vi "Agilent SNA Read Status Bytes.vi"(7 "Agilent SNA & SWP":T1, 8 "error in (no error)":errorcluster, 11 "VISA Resource Names":T2) -> (0 "error out":errorcluster, 1 "Extended Status Byte":bool[](array[boolean]), 2 "Status Byte":bool[](array[boolean]), 3 "dup VISA Resource Names":T2)   [LabVIEW 2011]
doc: "This VI for the HP8753B Network Analyzer reads the status byte and the two event status registers. The two status registers are read out as regular output and will therefore clear anything already in the output queue."
uses:
  TypeDefs/Agilent SNA VISA.ctl
  TypeDefs/Agilent SNA Instrument Info.ctl
panel:
  # "Self Test Failure\n\nOperation Failure\n\nKnob Activity\n\nAction Requested Not Possible\n\nLimit Test Failed\n\nFront Panel Preset or Power On\n\nDetector Uncal"
  # "Any Front Panel Key Pressed\n\nNumeric Entry Completed\n\nChange in Extended Status Byte\n\nSoftkey Only Pressed\n\nOperation Complete\n\nHP-IB Syntax Error\n\nRequest Service (SRQ)\n\nSweep Complete"
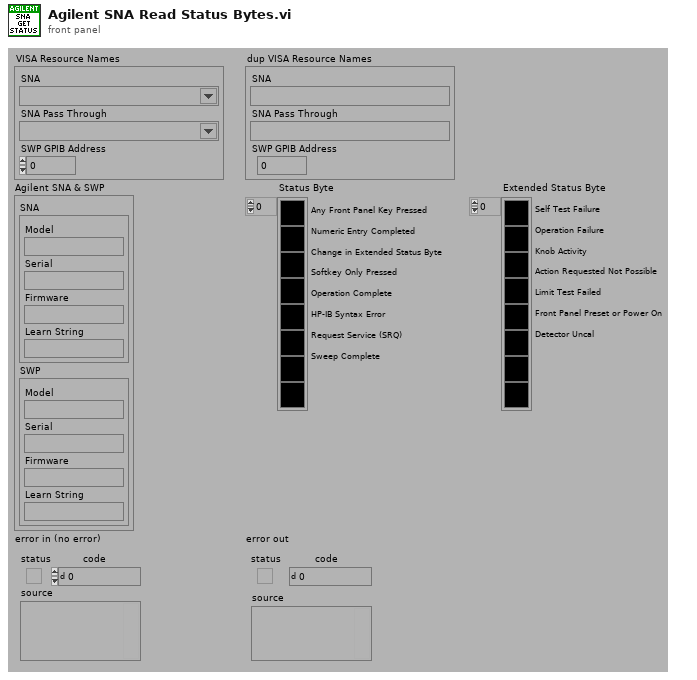
[diagram p1: front panel]
types:
  T1 = typedef "Agilent SNA Instrument Info.ctl" = cluster{"SNA":cluster{"Model":string, "Serial":string, "Firmware":string, "Learn String":string}, "SWP":cluster{"Model":string, "Serial":string, "Firmware":string, "Learn String":string}}
  T2 = typedef "Agilent SNA VISA.ctl" = cluster{"SNA":refnum<visa-resource-name>, "SNA Pass Through":refnum<visa-resource-name>, "SWP GPIB Address":i32}
  T3 = typedef "Agilent SNA Model.ctl" = enum16{"Not Supported", "8757X"}
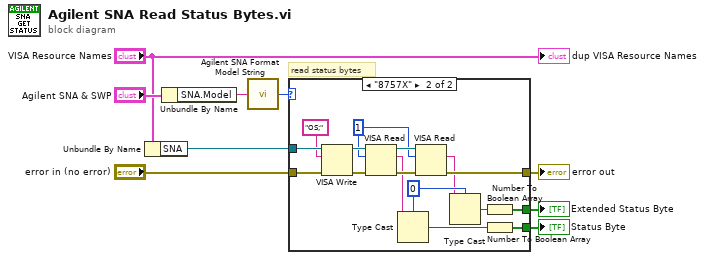
[diagram p0: block diagram]
diagram:
  # "read status bytes"
  n1 = Unbundle By Name("VISA Resource Names") -> ("SNA"=w3:refnum<visa-resource-name>)
  n2 = Unbundle By Name("Agilent SNA & SWP") -> ("SNA.Model"=w4:string)
  n3 = call "Agilent SNA Format Model String.vi"("Model String"=w4) -> ("Model"=w5:T3)
  n4 = case shown="\"8757X\"" w5 {
    tunnel: "error in (no error)" -> [w10 w26]
    tunnel: w3 -> [_ w25]
    tunnel: [_ w24] -> w8
    tunnel: [_ w23] -> w7
    tunnel: [w10 w18] -> w1
    frame "Not Supported" {
    }
    frame "8757X" {
      w12 = u8 0
      w16 = u32 1
      n5 = VISA Write(VISA resource name=w25, write buffer="OS;", error in (no error)=w26) -> (VISA resource name out=w21:refnum<visa-resource-name>, error out=w22:errorcluster)  [unwired: 1 out]
      n6 = VISA Read(VISA resource name=w21, byte count=w16, error in (no error)=w22) -> (VISA resource name out=w17:refnum<visa-resource-name>, read buffer=w15:string, error out=w19:errorcluster)  [unwired: 1 out]
      n7 = Type Cast(type=w12, x=w15) -> (*(type *) &x=w14:u8)
      n8 = VISA Read(VISA resource name=w17, byte count=w16, error in (no error)=w19) -> (read buffer=w11:string, error out=w18:errorcluster)  [unwired: 2 out]
      n9 = Type Cast(type=w12, x=w11) -> (*(type *) &x=w13:u8)
      n10 = Number To Boolean Array(number=w13) -> (Boolean array=w24:bool[])
      n11 = Number To Boolean Array(number=w14) -> (Boolean array=w23:bool[])
    }
  }
  "error out" <- w1
  "Extended Status Byte" <- w8
  "Status Byte" <- w7
  "dup VISA Resource Names" <- "VISA Resource Names"
